vi "Acquire Aquatrak Data.vi"(8 "Error In":errorcluster, 11 "Settings in":T1) -> (0 "Error Out":errorcluster, 1 "Aquatrak Data":string, 2 "Bytes at Serial Port":u32, 3 "Settings out":T1, 4 "Aquatrak Data Timestamp":timestamp format="%<%X  %x>T", 6 "cRIO Data Timestamp":timestamp format="%<%X  %x>T")   [LabVIEW 2019, in "cRIO Acquisition.lvlib"]
uses:
  cRIO Acquisition.lvlib
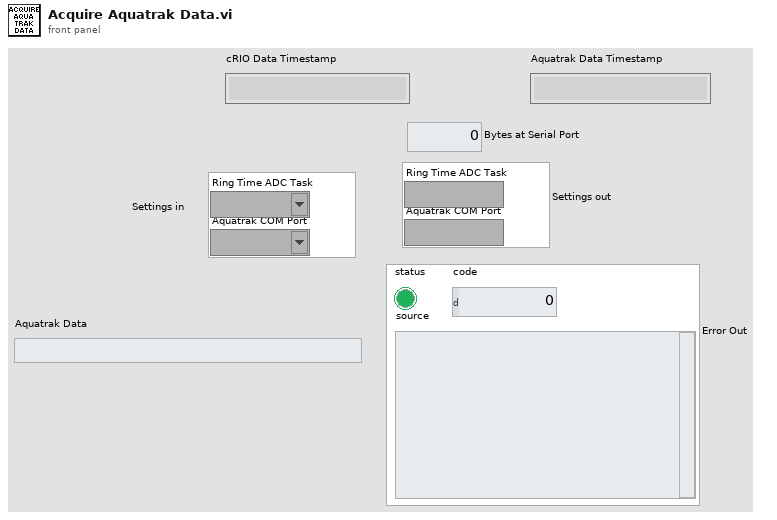
[diagram p1: front panel]
types:
  T1 = cluster{"Ring Time ADC Task":refnum<k21>, "Aquatrak COM Port":refnum<visa-resource-name>}
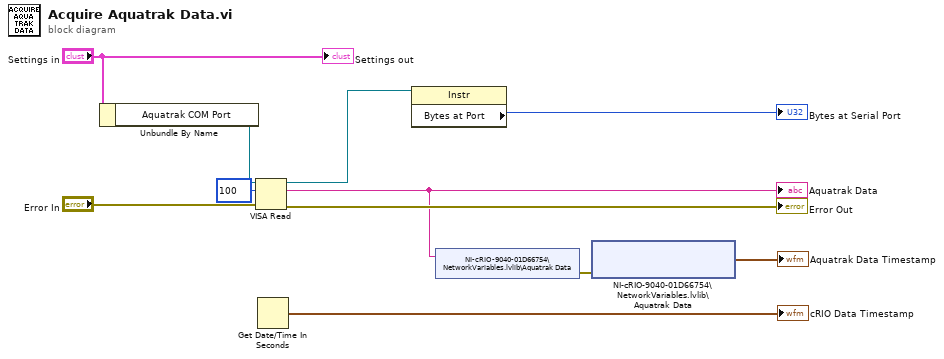
[diagram p0: block diagram]
diagram:
  n1 = Unbundle By Name("Settings in") -> ("Aquatrak COM Port"=w9:refnum<visa-resource-name>)
  n2 = VISA Read(VISA resource name=w9, byte count=u32 100, error in (no error)="Error In") -> (VISA resource name out=w7:refnum<visa-resource-name>, read buffer=w4:string, error out=→"Error Out":errorcluster)  [unwired: 1 out]
  "Aquatrak Data" <- w4
  n3 = Get Date/Time In Seconds() -> (seconds since 1Jan1904=→"cRIO Data Timestamp":timestamp)
  n4 = property class="Instr"(reference=w7) -> ("Bytes at Port"=→"Bytes at Serial Port":u32)  [unwired: 1 in, 2 out]
  n5 = shared-variable "NI-cRIO-9040-01D66754\\NetworkVariables.lvlib\\Aquatrak Data"(w4) -> (error out=w3:errorcluster)  [unwired: 1 in]
  n6 = shared-variable "NI-cRIO-9040-01D66754\\NetworkVariables.lvlib\\Aquatrak Data"(error in=w3) -> (→"Aquatrak Data Timestamp":timestamp)  [unwired: 2 out]
  "Settings out" <- "Settings in"
